vi "delta bulid.vi"(6 "reset data":bool, 7 "first side":bool, 8 "mean factor":dbl=-40.0 format="%#_13g", 10 "new data":T2, 11 "memory data":T1) -> (0 "amp cal":cluster{"freqency":dbl[], "Array":dbl[]}, 1 "phase cal":cluster{"freqency":dbl[], "Array":dbl[]}, 3 "delta splitter":T1)   [LabVIEW 2021]
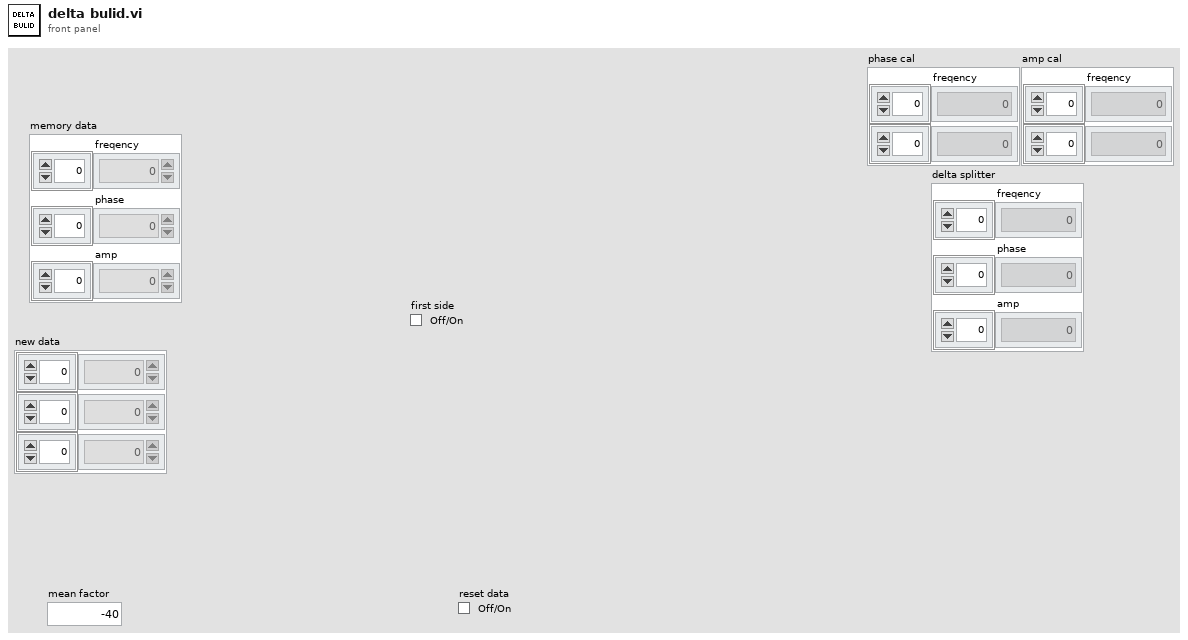
[diagram p1: front panel]
types:
  T1 = cluster{"freqency":dbl[], "phase":dbl[], "amp":dbl[]}
  T2 = cluster{"Array":dbl[], "Array":dbl[], "Array":dbl[]}
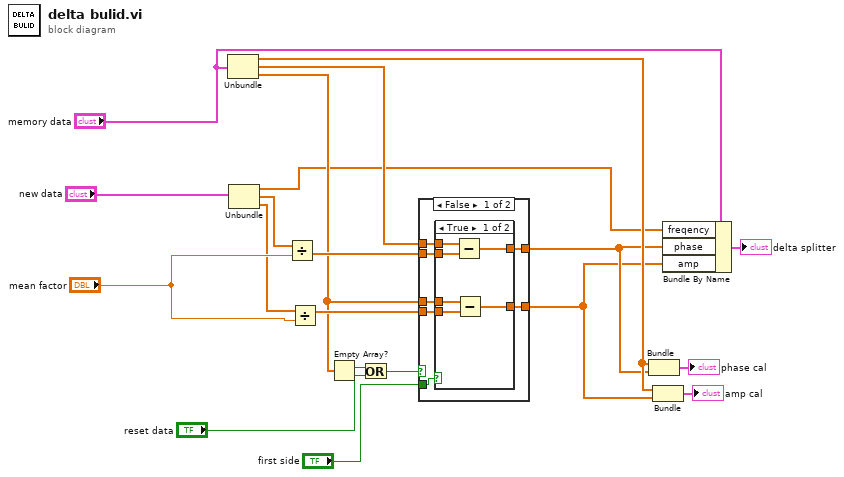
[diagram p0: block diagram]
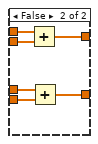
[diagram p2: hidden frame]
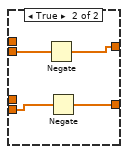
[diagram p3: hidden frame]
diagram:
  n1 = Unbundle("memory data") -> ("freqency"=w14:dbl[], "phase"=w18:dbl[], "amp"=w9:dbl[])
  n2 = Unbundle("new data") -> ("Array"=w7:dbl[], "Array"=w20:dbl[], "Array"=w15:dbl[])
  n3 = Divide(x=w20, y="mean factor") -> (x/y=w19:dbl[])
  n4 = Divide(x=w15, y="mean factor") -> (x/y=w17:dbl[])
  n5 = Empty Array?(array=w9) -> (empty?=w6:bool)
  n6 = Or(x=w6, y="reset data") -> (x .or. y?=w4:bool)
  n7 = case shown="False" w4 {
    tunnel: w19 -> [w27 w43]
    tunnel: w18 -> [w26 _]
    tunnel: w17 -> [w25 w41]
    tunnel: [w24 w42] -> w13
    tunnel: [w23 w40] -> w12
    tunnel: w9 -> [w22 _]
    tunnel: "first side" -> [w21 _]
    frame False {
      n8 = case shown="True" w21 {
        tunnel: w27 -> [w33 w39]
        tunnel: w26 -> [w32 w38]
        tunnel: w25 -> [w31 w37]
        tunnel: [w30 w36] -> w24
        tunnel: [w29 w35] -> w23
        tunnel: w22 -> [w28 w34]
        frame True {
          n9 = Subtract(x=w32, y=w33) -> (x-y=w30:dbl[])
          n10 = Subtract(x=w28, y=w31) -> (x-y=w29:dbl[])
        }
        frame False {
          n11 = Add(x=w38, y=w39) -> (x+y=w36:dbl[])
          n12 = Add(x=w34, y=w37) -> (x+y=w35:dbl[])
        }
      }
    }
    frame True {
      n13 = Negate(x=w43) -> (-x=w42:dbl[])
      n14 = Negate(x=w41) -> (-x=w40:dbl[])
    }
  }
  n15 = Bundle("freqency"=w14, w13) -> (→"phase cal":cluster{"freqency":dbl[], dbl[]})  [unwired: 1 in]
  n16 = Bundle("freqency"=w14, w12) -> (→"amp cal":cluster{"freqency":dbl[], dbl[]})  [unwired: 1 in]
  n17 = Bundle By Name(cluster="memory data", "freqency"=w7, "phase"=w13, "amp"=w12) -> (→"delta splitter":T1)
